vi "DMM Engine.vi"() -> ()   [LabVIEW 2011]
uses:
  Tushars Events/Software/Modules/EventClient_ObjectReference.ctl
  Strict Type Controls/Settings Operation.ctl
  <vilib>/Instr/_visa.llb/VISA Configure Serial Port (Instr).vi
panel:
  out "Quit":bool
  out "error out":errorcluster
  in  "error in (no error)":errorcluster
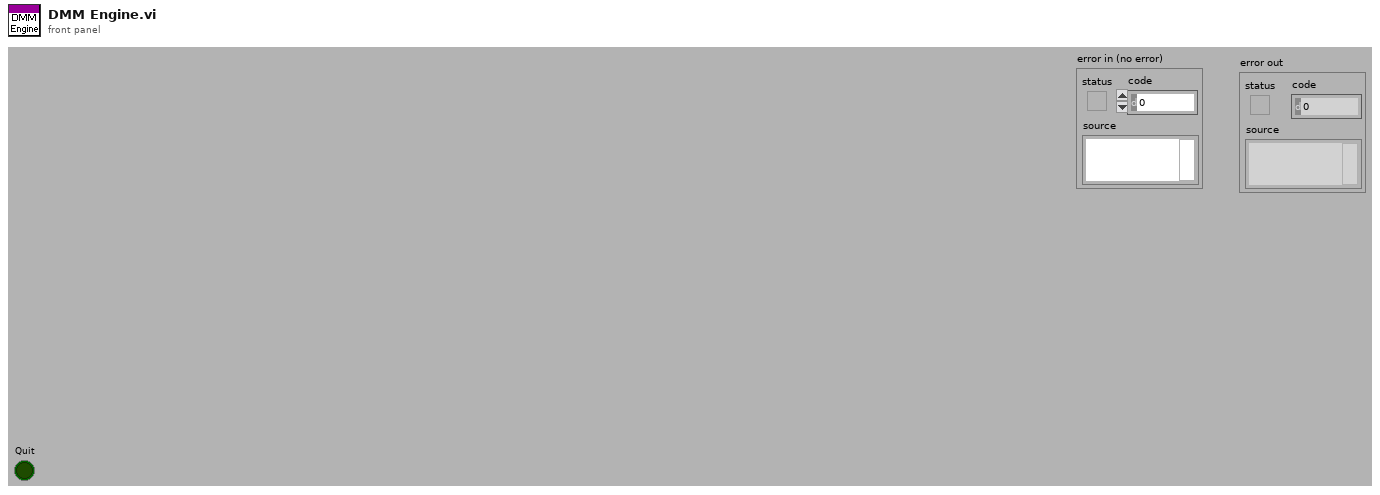
[diagram p1: front panel]
types:
  T1 = typedef "EventClient_ObjectReference.ctl" = refnum<k1>
  T2 = typedef "Settings Operation.ctl" = enum8{"Get Value", "Set Value", "Read File", "Write File", "Write Stored Value"}
  T3 = typedef "Settings.ctl" = cluster{"DMM Settings":cluster{"Port":refnum<visa-resource-name>, "baud rate":u32, "data bits":u16, "stop bits":u16, "parity":enum16{"None", "Odd", "Even", "Mark", "Space"}, "flow control":enum16{"None", "XON/XOFF", "RTS/CTS", "XON/XOFF & RTS/CTS", "DTR/DSR", "XON/XOFF & DTR/DSR"}}, "Modbus Settings":cluster{"Port":refnum<visa-resource-name>, "baud rate":u32, "parity":enum16{"None", "Odd", "Even", "Mark", "Space"}, "flow control":enum16{"None", "XON/XOFF", "RTS/CTS", "XON/XOFF & RTS/CTS", "DTR/DSR", "XON/XOFF & DTR/DSR"}}}
  T4 = enum16{"None", "XON/XOFF", "RTS/CTS", "XON/XOFF & RTS/CTS", "DTR/DSR", "XON/XOFF & DTR/DSR"}
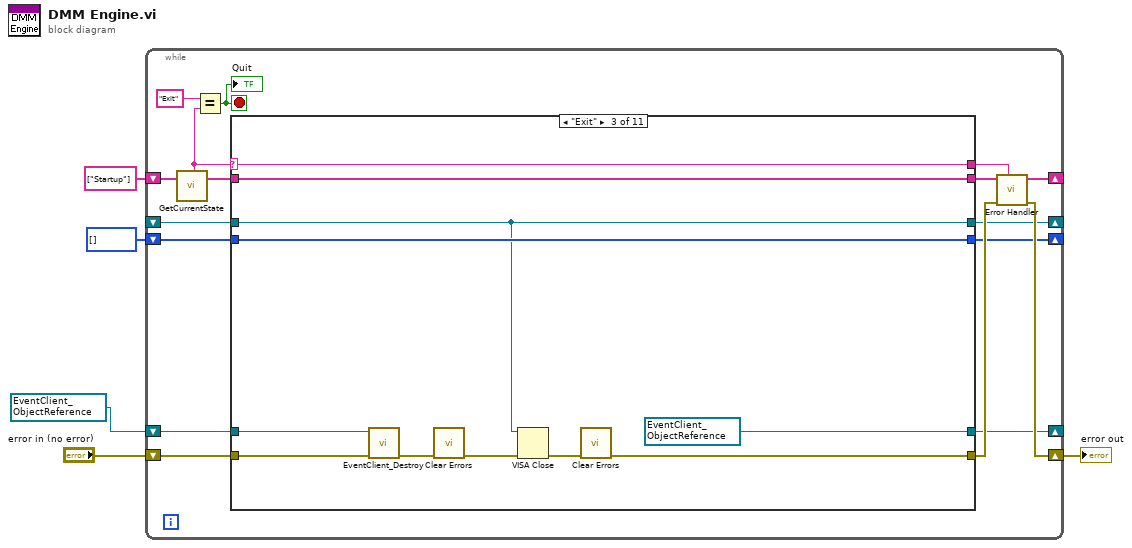
[diagram p0: block diagram]
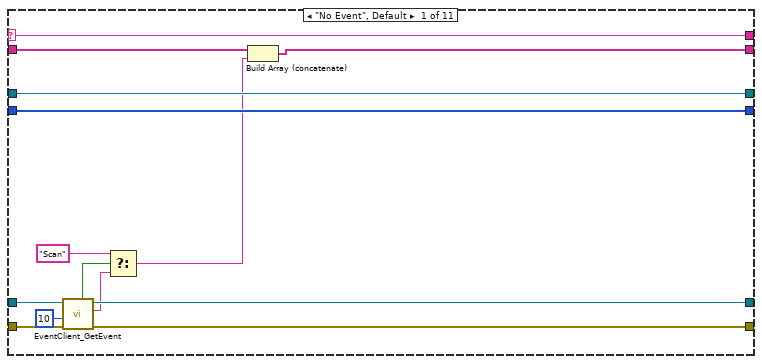
[diagram p2: hidden frame]
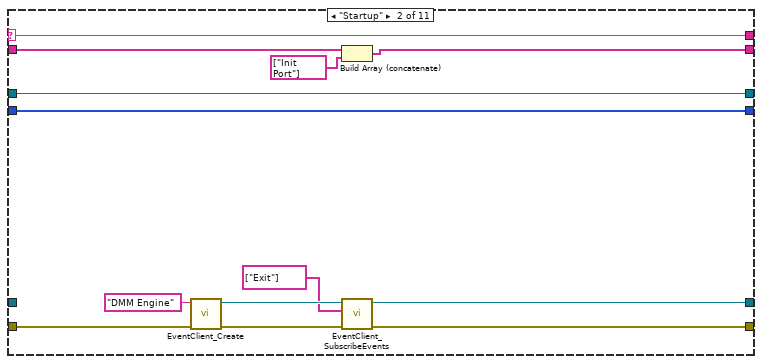
[diagram p3: hidden frame]
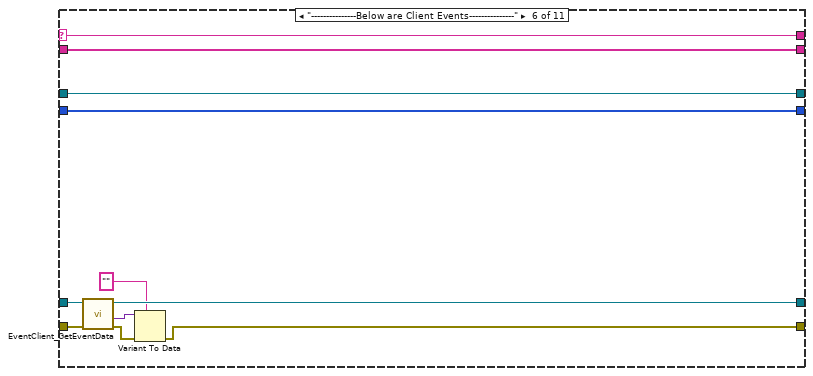
[diagram p6: hidden frame]
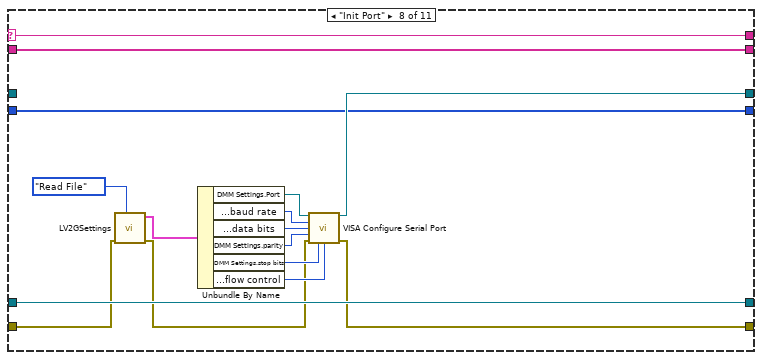
[diagram p8: hidden frame]
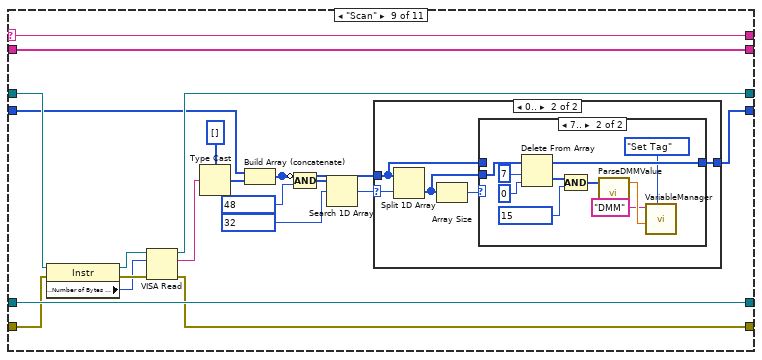
[diagram p9: hidden frame]
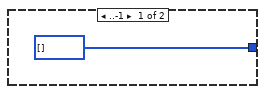
[diagram p10: hidden frame]
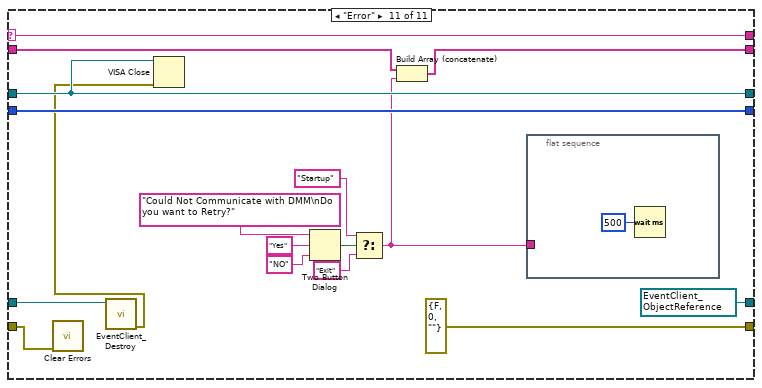
[diagram p13: hidden frame]
diagram:
  w2 = T1 refnum items=["EventClient"] ("reference")
  n1 = while {
    shift-right: [w18] -> _
    shift-left: string[] ["Startup"] ("State Array Out") -> [w22]
    shift-right: [w14] -> w3
    shift-left: "error in (no error)" -> [w15]
    shift-right: [w11] -> _
    shift-left: w2 -> [w10]
    shift-right: [w9] -> _
    shift-left: _ -> [w8]
    shift-right: [w6] -> _
    shift-left: u8[] [] -> [w7]
    stop <- w19 stop-if-true
    n2 = call "GetCurrentState.vi"("State Array In"=w22) -> ("Current State"=w12:string, "State Array Out"=w21:string[])  [unwired: 1 in, 16 out]
    n3 = Equal?(x="Exit", y=w12) -> (x = y?=w19:bool)
    "Quit" <- w19
    n4 = case shown="\"Exit\"" w12 {
      selector: w12 -> [w36 w49 w60 w65 w71 w82 w88 w104 w124 w148 w165]
      tunnel: w21 -> [w29 w48 w59 w66 w72 w83 w89 w105 w125 w147 w161]
      tunnel: [w31 w47 w59 w66 w72 w83 w89 w105 w125 w147 w160] -> w17
      tunnel: [w33 w43 w50 w64 w70 w78 w87 w93 w106 w146 errorcluster {"status"=FALSE, "code"=0, "source"=""} ("error in (no error)")] -> w13
      tunnel: [w36 w49 w60 w65 w71 w82 w88 w104 w124 w148 w165] -> w16
      tunnel: w15 -> [w34 w45 w57 w64 w70 w80 w87 w102 w107 w146 w150]
      tunnel: [w32 w41 w56 w63 w69 w76 w86 w103 w123 w145 w151] -> w11
      tunnel: w10 -> [w35 _ w58 w63 w69 w81 w86 w103 w123 w145 w152]
      tunnel: [w28 w38 w54 w62 w68 w75 w85 w92 w110 w144 w162] -> w9
      tunnel: w8 -> [w28 w38 w54 w62 w68 w75 w85 _ w111 w144 w162]
      tunnel: w7 -> [w27 w37 w55 w61 w67 w74 w84 w91 w109 w143 w163]
      tunnel: [w27 w37 w55 w61 w67 w74 w84 w91 w108 w143 w163] -> w6
      frame "No Event", Default {
        n5 = call "EventClient_GetEvent.vi"("error in (no error)"=w34, "timeout in ms (-1)"=10, "reference"=w35) -> ("error out"=w33:errorcluster, "Name"=w24:string, "reference out"=w32:T1, "timed out?"=w26:bool)  [unwired: 5 out]
        n6 = Select(t="Scan" ("x"), s=w26, f=w24) -> (s? t:f=w23:string)
        n7 = Build Array (concatenate)(w29, w23) -> (w31:string[])
      }
      frame "Startup" {
        n8 = call "EventClient_Create.vi"("error in (no error)"=w45, "Instance Name"="DMM Engine") -> ("error out"=w44:errorcluster, "reference"=w42:T1)  [unwired: 8 out]
        n9 = Build Array (concatenate)(w48, string[] ["Init Port"] ("State Array Out")) -> (w47:string[])
        n10 = call "EventClient_SubscribeEvents.vi"("error in (no error)"=w44, "Events"=string[] ["Exit"], "reference"=w42) -> ("error out"=w43:errorcluster, "reference out"=w41:T1)  [unwired: 7 out]
      }
      frame "Exit" {
        w56 = T1 refnum items=["EventClient"] ("reference out")
        n11 = call "EventClient_Destroy.vi"("error in (no error)"=w57, "reference"=w58) -> ("error out"=w53:errorcluster)  [unwired: 9 out]
        n12 = call <vilib>:"Clear Errors.vi"("error in (no error)"=w53) -> ("error out"=w52:errorcluster)  [unwired: 6 out]
        n13 = VISA Close(VISA resource name=w54, error in (no error)=w52) -> (error out=w51:errorcluster)
        n14 = call <vilib>:"Clear Errors.vi"("error in (no error)"=w51) -> ("error out"=w50:errorcluster)  [unwired: 6 out]
      }
      frame "---------------Below are UI Events---------------" {
        # "This State will never Execute\nIt is added just for improving code readability please do not remove this case"
      }
      frame "---------------Below are Menu Events---------------" {
        # "This State will never Execute\nIt is added just for improving code readability please do not remove this case"
      }
      frame "---------------Below are Client Events---------------" {
        n15 = call "EventClient_GetEventData.vi"("error in (no error)"=w80, "reference"=w81) -> ("error out"=w79:errorcluster, "Data"=w77:variant, "reference out"=w76:T1)  [unwired: 7 out]
        n16 = Variant To Data(error in=w79, type="", Variant=w77) -> (error out=w78:errorcluster)  [unwired: 1 out]
      }
      frame "---------------Below are Subroutine states---------------" {
      }
      frame "Init Port" {
        n17 = call "LV2GSettings.vi"("Operation"=Settings_Operation."Read File", "error in (no error)"=w102) -> ("error out"=w94:errorcluster, "Settings out"=w100:T3)  [unwired: 1 in, 7 out]
        n18 = Unbundle By Name(w100) -> ("DMM Settings.Port"=w90:refnum<visa-resource-name>, "DMM Settings.baud rate"=w99:u32, "DMM Settings.data bits"=w98:u16, "DMM Settings.parity"=w97:enum16{"None", "Odd", "Even", "Mark", "Space"}, "DMM Settings.stop bits"=w96:u16, "DMM Settings.flow control"=w95:T4)
        n19 = call-poly "VISA Configure Serial Port"("VISA resource name"=w90, "baud rate (9600)"=w99, "data bits (8)"=w98, "parity (0:none)"=w97, "error in (no error)"=w94, "stop bits (10: 1 bit)"=w96, "flow control (0:none)"=w95) -> ("VISA resource name out"=w92:refnum<visa-resource-name>, "error out"=w93:errorcluster)  [unwired: 7 out]
      }
      frame "Scan" {
        n20 = property class="Instr"(reference=w111, error in=w107) -> (reference out=w112:refnum<visa-resource-name>, error out=w122:errorcluster, "Serial Settings:Number of Bytes at Serial Port"=w113:u32)
        n21 = VISA Read(VISA resource name=w112, byte count=w113, error in (no error)=w122) -> (VISA resource name out=w110:refnum<visa-resource-name>, read buffer=w114:string, error out=w106:errorcluster)  [unwired: 1 out]
        n22 = Type Cast(type=u8[] [], x=w114) -> (*(type *) &x=w120:u8[])
        n23 = Build Array (concatenate)(w109, w120) -> (w119:u8[])
        n24 = Compound Arithmetic op=AND(invert w119, u8 48) -> (w116:u8[])
        n25 = Search 1D Array(1D array=w116, element=u8 32) -> (index of element=w118:i32)  [unwired: 1 out]
        n26 = case shown="0.." w118 {
          selector: w118 -> [_ w131]
          tunnel: [u8[] [] w129] -> w108
          tunnel: w119 -> [_ w128]
          frame ..-1 {
          }
          frame 0.. {
            n27 = Split 1D Array(array=w128, index=w131) -> (second subarray=w127:u8[])  [unwired: 1 out]
            n28 = Array Size(array=w127) -> (size(s)=w130:i32)
            n29 = case shown="7.." w130 {
              tunnel: [w132 w137] -> w129
              tunnel: w128 -> [w132 _]
              tunnel: w127 -> [_ w142]
              frame 0, Default {
              }
              frame 7.. {
                n30 = Delete From Array(array=w142, length=7, index=0) -> (deleted portion=w136:u8[], array with subset deleted=w137:u8[])
                n31 = Compound Arithmetic op=AND(w136, u8 15) -> (w139:u8[])
                n32 = call "ParseDMMValue.vi"("DMM Data"=w139) -> ("Value"=w135:dbl)  [unwired: 4 out]
                n33 = call "VariableManager.vi"("Operation"=enum16{"Get Tag", "Set Tag"}."Set Tag", "Value"=w135, "Tag"="DMM") -> ()  [unwired: 9 out]
              }
            }
          }
        }
      }
      frame "---------------Below are Error Handling VIs---------------" {
      }
      frame "Error" {
        w151 = T1 refnum items=["EventClient"] ("reference")
        n34 = call <vilib>:"Clear Errors.vi"("error in (no error)"=w150) -> ()  [unwired: 7 out]
        n35 = call "EventClient_Destroy.vi"("reference"=w152) -> ("error out"=w149:errorcluster)  [unwired: 1 in, 9 out]
        n36 = VISA Close(VISA resource name=w162, error in (no error)=w149) -> ()  [unwired: 1 out]
        n37 = Two Button Dialog(message="Could Not Communicate with DMM\nDo you want to Retry?", 1:"NO" ("F button name (\"Cancel\")"), 2:"Yes" ("T button name (\"OK\")")) -> (T button?=w156:bool)
        n38 = Select(t="Startup" ("String"), s=w156, f="Exit" ("String")) -> (s? t:f=w153:string)
        n39 = Build Array (concatenate)(w161, w153) -> (w160:string[])
        n40 = flat-sequence {
          tunnel: w153 -> [_]
          frame #0 {
            n41 = Wait (ms)(milliseconds to wait=u32 500) -> ()  [unwired: 1 out]
          }
        }
      }
    }
    n42 = call "Error Handler.vi"("Current State"=w16, "error in (no error)"=w13, "Msg Queue In"=w17) -> ("error out"=w14:errorcluster, "Msg Queue Out"=w18:string[])  [unwired: 1 in, 6 out]
  }
  "error out" <- w3
